vi "Construct.vi"(1 "Canvas Ref in":refnum<vi>, 2 "Collsion Cell Size":i16, 3 "Target Frame Rate":i8) -> (0 "PhysicsSystem out":refnum<class "PhysicsSystem.lvclass">)   [LabVIEW 2022 SP3, in "PhysicsSystem.lvclass"]
uses:
  PhysicsSystem.lvclass
  PhysicsSystem.lvclass/PhysicsSystem.ctl
  Math/Vector2/Vector2.lvclass
  Objects/Collisions/CollisionGrid/CollisionGrid.lvclass
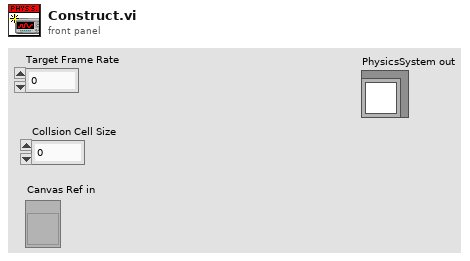
[diagram p1: front panel]
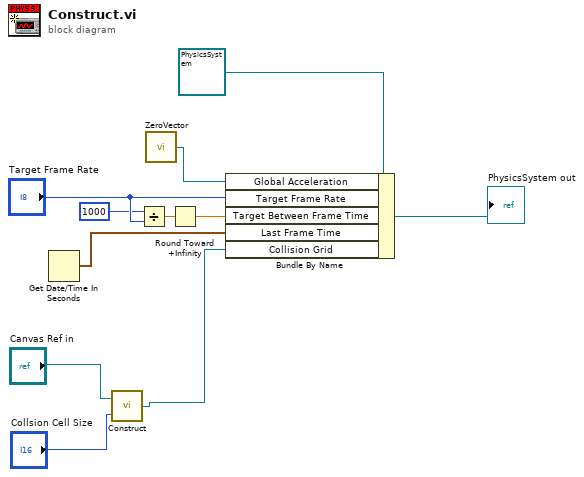
[diagram p0: block diagram]
diagram:
  n1 = Get Date/Time In Seconds() -> (seconds since 1Jan1904=w4:timestamp)
  n2 = call "Construct.vi"("Cell Size"="Collsion Cell Size", "Canvas Ref in"="Canvas Ref in") -> ("CollisionGrid.lvclass"=w1:refnum<class "CollisionGrid.lvclass">)
  n3 = Divide(x=1000, y="Target Frame Rate") -> (x/y=w9:dbl)
  n4 = call "ZeroVector.vi"() -> ("Zero Vector"=w5:refnum<class "Vector2.lvclass">)
  n5 = Round Toward +Infinity(x=w9) -> (ceil(x): smallest int >= x=w8:dbl)
  n6 = Bundle By Name(cluster=refnum<class "PhysicsSystem.lvclass"> refnum ("PhysicsSystem.lvclass"), "Global Acceleration"=w5, "Target Frame Rate"="Target Frame Rate", "Target Between Frame Time"=w8, "Last Frame Time"=w4, "Collision Grid"=w1) -> (→"PhysicsSystem out":refnum<class "PhysicsSystem.lvclass">)
